vi "Create.vi"(8 "error in (no error)":errorcluster) -> (0 "error out":errorcluster, 3 "Builder out":refnum<class "Builder.lvclass">)   [LabVIEW 2020, in "Builder Tools.lvlib" / "Builder.lvclass"]
uses:
  Builder.lvclass
  Builder.lvclass/Builder.ctl
  Build Events API/Build Events API.lvclass
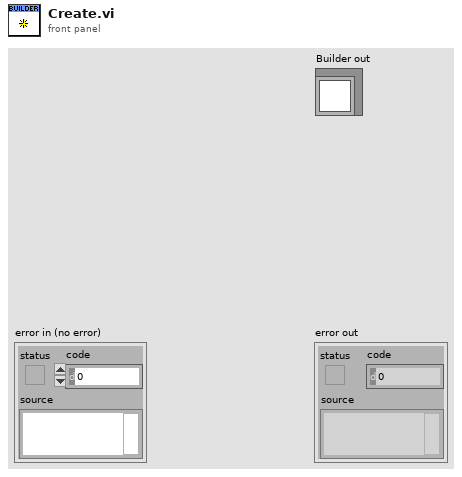
[diagram p1: front panel]
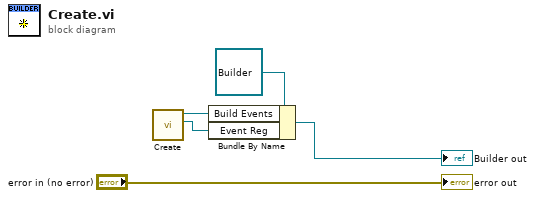
[diagram p0: block diagram]
diagram:
  n1 = call "Create.vi"() -> ("Event Reg"=w1:refnum<event-registration>, "Build Events API out"=w2:refnum<class "Build Events API.lvclass">)  [unwired: 9 in, 1 out]
  n2 = Bundle By Name(cluster=refnum<class "Builder.lvclass"> refnum ("Builder in"), "Build Events"=w2, "Event Reg"=w1) -> (→"Builder out":refnum<class "Builder.lvclass">)
  "error out" <- "error in (no error)"
